vi "Build MAP from base64 table.vi"() -> ()   [LabVIEW 2021]
uses:
  <vilib>/Utility/file.llb/Read Delimited Spreadsheet (string).vi
panel:
  out "Map":map{string, u8}(c390)
  out "element 2":string
  out "element":string
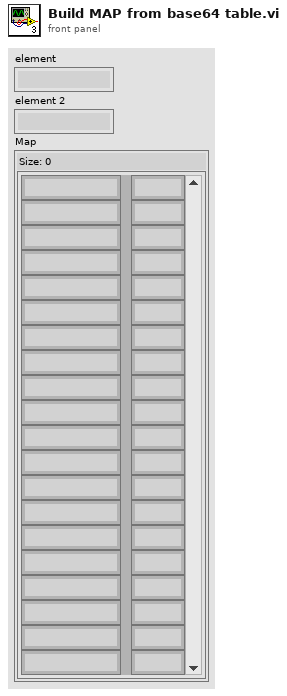
[diagram p1: front panel]
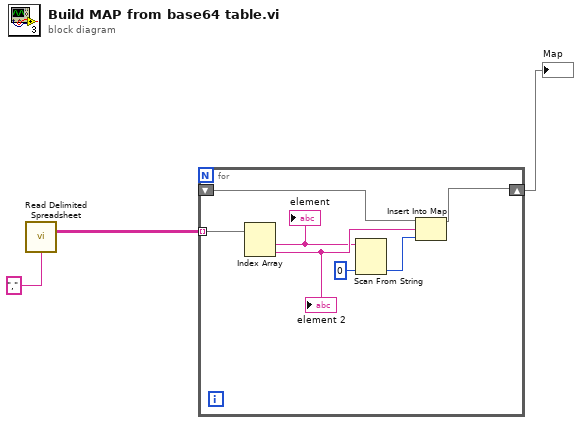
[diagram p0: block diagram]
diagram:
  n1 = call-poly <vilib>:"Read Delimited Spreadsheet.vi"("delimiter (\\t)"="," ("delimiter (\\t)")) -> ("all rows"=w2:string[][])  [unwired: 9 in, 5 out]
  n2 = for {
    tunnel: w2 -> [w10] mode=indexing
    shift-right: [w9] -> w1
    shift-left: _ -> [w8]
    n3 = Index Array(array=w10) -> (element #1=w6:string, element #2=w7:string)  [unwired: 2 in]
    "element" <- w6
    "element 2" <- w7
    n4 = Scan From String(input string=w6, default 1=u8 0 ("default value 1")) -> (output 1=w4:u8)  [unwired: 3 in, 3 out]
    n5 = Insert Into Map(map in=w8, key=w7, value=w4) -> (map out=w9:map{string, u8})  [unwired: 2 out]
  }
  "Map" <- w1
